vi "NHQ203M Read.vi"(3 "error in (no error)":errorcluster, 4 "Write Command":string="*RST;FORM:ELEM READ;:DISP:ENAB 0;:CURR:RANG:AUTO 1;*IDN?", 5 "VISA resource name":refnum<visa-resource-name>) -> (0 "Error out":errorcluster, 1 "Feedback":string, 2 "VISA out":refnum<visa-resource-name>)   [LabVIEW 2018]
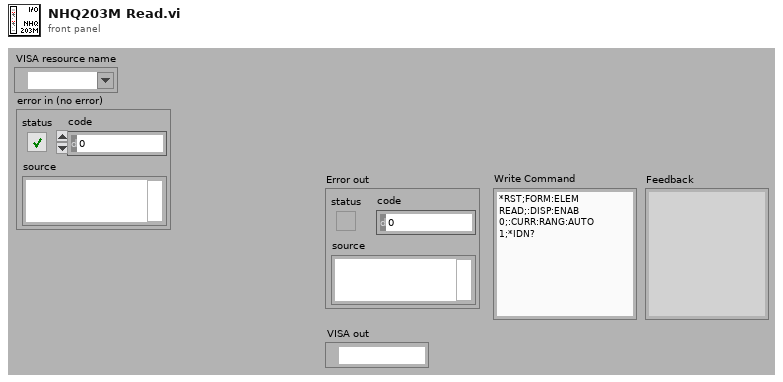
[diagram p1: front panel]
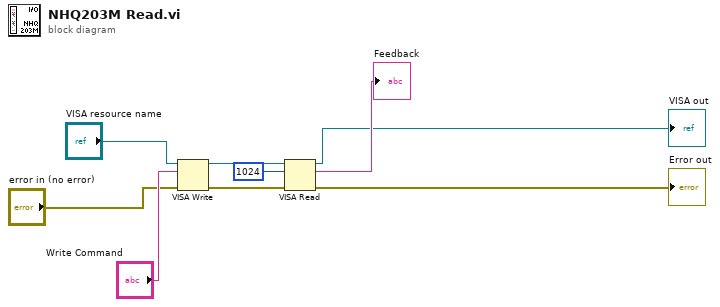
[diagram p0: block diagram]
diagram:
  n1 = VISA Write(VISA resource name="VISA resource name", write buffer="Write Command", error in (no error)="error in (no error)") -> (VISA resource name out=w8:refnum<visa-resource-name>, error out=w7:errorcluster)  [unwired: 1 out]
  n2 = VISA Read(VISA resource name=w8, byte count=u32 1024, error in (no error)=w7) -> (VISA resource name out=→"VISA out":refnum<visa-resource-name>, read buffer=→"Feedback":string, error out=→"Error out":errorcluster)  [unwired: 1 out]
